vi "Example - Download with Progress and Abort.vi"() -> ()   [LabVIEW 2019]
uses:
  <vilib>/httpClient/LabVIEWHTTPClient.lvlib
  Get Async.lvlib
  <vilib>/Utility/sysdir.llb/System Directory Type.ctl
  HTTP Client Extensions.lvlib
panel:
  out "Rediect URLs":string[](array[string])
  in  "timeout (10000)":i32=10000
  out "complete":bool[](array[boolean])
  in  "Exit":bool
  in  "Start":bool
  in  "Files to Download":string[](array[string])=["http://download.ni.com/evaluation/labview/lvtn/vipm/packages/NI_GDS_2016/NI_GDS_2016-1.1.83.83.vip", "http://download.ni.com/evaluation/labview/lvtn/vipm/packages/ni_gds/ni_gds-1.1.87.94.vip", "http://download.ni.com/evaluation/labview/lvtn/vipm/packages/s5s_aloha/s5s_aloha-2.0.0.22.vip", "http://download.ni.com/evaluation/labview/lvtn/vipm/packages/s5s_aloha_system/s5s_aloha_system-2.0.0.22.vip"]
  out "Progress":dbl[](array[slide]) scale=0.0..100.0
  out "bytes downloaded":i64[](array[numeric])
  out "file size (bytes)":i64[](array[numeric])
  in  "Abort":bool
  in  "Folder to save file(s)":path
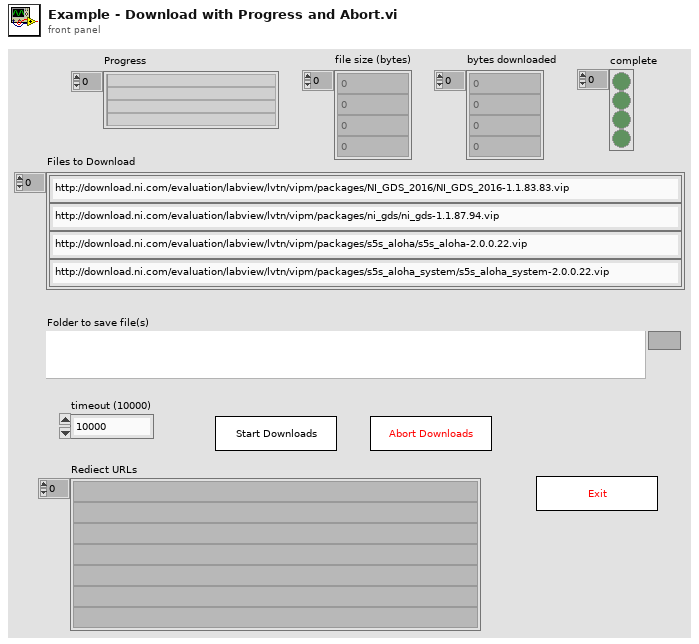
[diagram p1: front panel]
types:
  T1 = typedef "System Directory Type.ctl" = i32
  T2 = typedef "LabVIEWHTTPClient.lvlib/ClientHandle.ctl" = refnum<k1>
  T3 = typedef "HTTP Client Extensions.lvlib/Get Async.lvlib/Refnum Type.ctl" = refnum<k1>
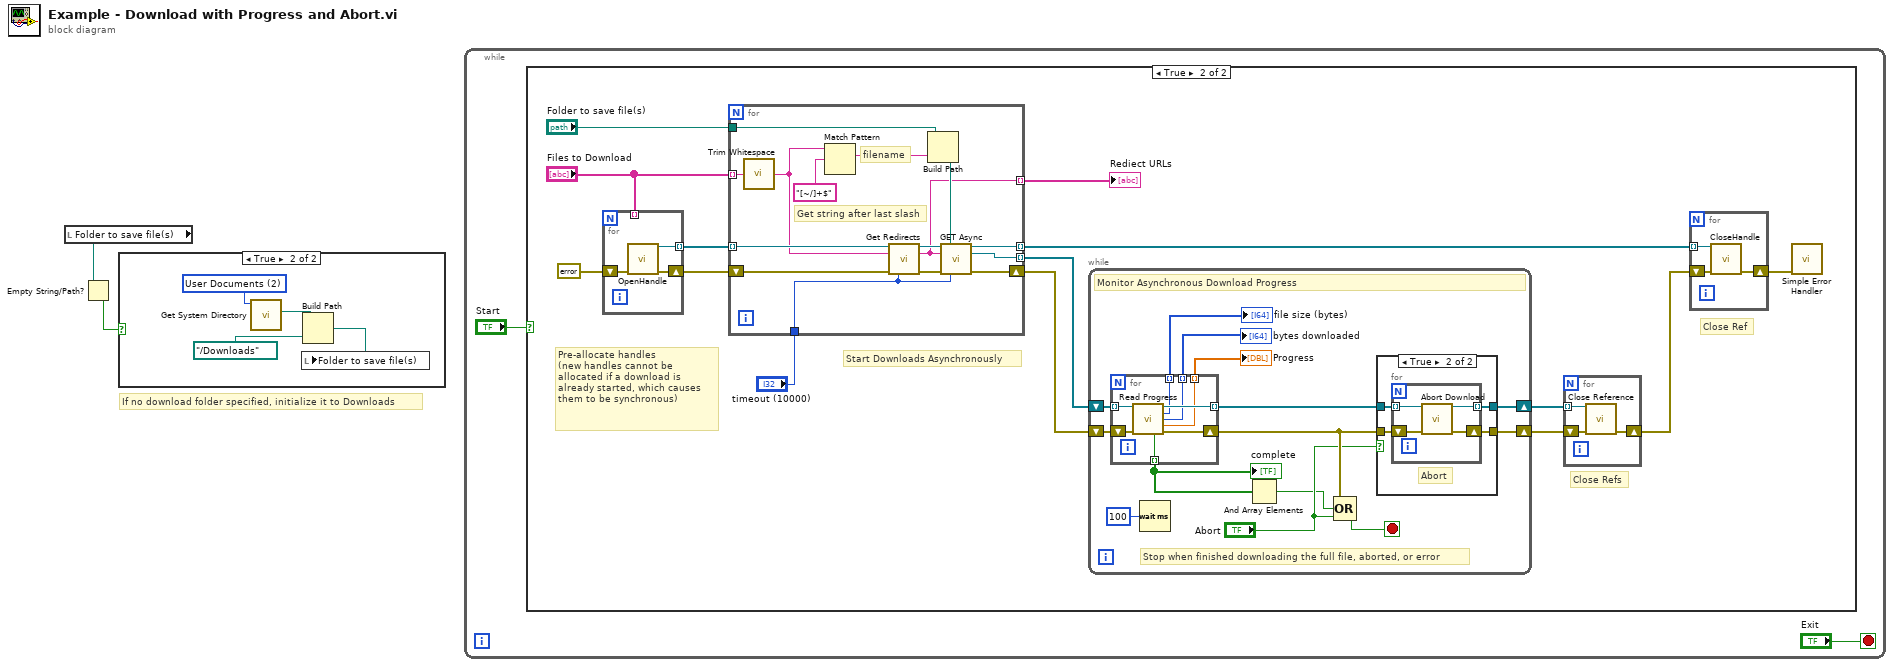
[diagram p0: block diagram]
diagram:
  # "If no download folder specified, initialize it to Downloads"
  n1 = local read "Folder to save file(s)"() -> (w2:path)
  n2 = Empty String/Path?(string/path=w2) -> (empty?=w1:bool)
  n3 = case shown="True" w1 {
    frame False {
    }
    frame True {
      w6 = T1 2 items=["User Home"=0, "User Desktop"=1, "User Documents"=2, "User Application Data"=3, "User Preferences"=4, "User Temporary"=5, "Public Documents"=6, "Public Application Data"=7, "Public Preferences"=8, "Public Cache"=13, "System Core Libraries"=9, "System Installed Libraries"=10, "Application Files"=11, "Boot Volume Root"=12] ("system directory type")
      n4 = call <vilib>:"Get System Directory.vi"("system directory type"=w6) -> ("system directory"=w5:path)  [unwired: 10 in]
      n5 = Build Path(base path=w5, name or relative path=path "../Downloads" ("base path")) -> (appended path=w3:path)
      n6 = local write "Folder to save file(s)"(w3) -> ()
    }
  }
  n7 = while {
    stop <- "Exit" stop-if-true
    n8 = case shown="True" "Start" {
      frame False {
      }
      frame True {
        # "Start Downloads Asynchronously"
        # "Close Ref"
        # "Close Refs"
        # "Pre-allocate handles\n(new handles cannot be allocated if a download is already started, which causes them to be synchronous)"
        n9 = for {
          shift-right: [w24] -> w14
          shift-left: errorcluster {"status"=FALSE, "code"=0, "source"=""} ("error out") -> [w25]
          tunnel: [w23] -> w13 mode=indexing
          tunnel: "Files to Download" -> [_] mode=indexing
          n10 = call <vilib>:"OpenHandle.vi"("error in (no error)"=w25) -> ("client handle out"=w23:T2, "error out"=w24:errorcluster)  [unwired: 13 in]
        }
        n11 = for {
          tunnel: "Folder to save file(s)" -> [w44]
          tunnel: [w41] -> w16 mode=indexing
          tunnel: "Files to Download" -> [w39] mode=indexing
          shift-right: [w42] -> w21
          shift-left: w14 -> [w34]
          tunnel: [w40] -> w20 mode=indexing
          tunnel: w13 -> [w37] mode=indexing
          tunnel: "timeout (10000)" -> [w33]
          tunnel: [w32] -> w9 mode=indexing
          # "Get string after last slash"
          # "filename"
          n12 = call <vilib>:"Trim Whitespace.vi"("string"=w39) -> ("trimmed string"=w36:string)  [unwired: 1 in]
          n13 = Match Pattern(string=w36, regular expression="[~/]+$") -> (match substring=w45:string)  [unwired: 1 in, 3 out]
          n14 = call "Get Redirects.vi"("client handle"=w37, "url"=w36, "error in (no error)"=w34, "timeout (10000)"=w33) -> ("client handle out"=w38:T2, "url out"=w32:string, "error out"=w35:errorcluster)  [unwired: 5 in, 4 out]
          n15 = Build Path(base path=w44, name or relative path=w45) -> (appended path=w43:path)
          n16 = call "GET Async.vi"("client handle"=w38, "output file"=w43, "url"=w32, "error in (no error)"=w35, "timeout (10000)"=w33) -> ("client handle out"=w40:T2, "get async handle"=w41:T3, "error out"=w42:errorcluster)  [unwired: 7 in, 1 out]
        }
        "Rediect URLs" <- w9
        n17 = while {
          shift-right: [w57] -> w18
          shift-left: w21 -> [w58]
          shift-right: [w53] -> w19
          shift-left: w16 -> [w59]
          stop <- w60 stop-if-true
          # "Stop when finished downloading the full file, aborted, or error"
          # "Monitor Asynchronous Download Progress"
          n18 = for {
            tunnel: w59 -> [w68] mode=indexing
            tunnel: [w61] -> w52 mode=indexing
            tunnel: [w62] -> w51 mode=indexing
            tunnel: [w65] -> w54 mode=indexing
            tunnel: [w64] -> w48 mode=indexing
            tunnel: [w63] -> w50 mode=indexing
            shift-right: [w66] -> w56
            shift-left: w58 -> [w67]
            n19 = call "Read Progress.vi"("HTTP GET Async handle"=w68, "error in (no error)"=w67) -> ("HTTP GET Async handle out"=w65:T3, "file size"=w62:i64, "bytes downloaded"=w61:i64, "percent complete"=w64:dbl, "download complete"=w63:bool, "error out"=w66:errorcluster)  [unwired: 8 in]
          }
          "bytes downloaded" <- w52
          "file size (bytes)" <- w51
          "Progress" <- w48
          "complete" <- w50
          n20 = Wait (ms)(milliseconds to wait=u32 100) -> ()  [unwired: 1 out]
          n21 = And Array Elements(Boolean array=w50) -> (logical AND=w49:bool)
          n22 = Compound Arithmetic op=OR(w56, w49, "Abort") -> (w60:bool)
          n23 = case shown="True" "Abort" {
            tunnel: [w70 w74] -> w57
            tunnel: w56 -> [w70 w73]
            tunnel: w54 -> [w69 w72]
            tunnel: [w69 w71] -> w53
            frame False {
            }
            frame True {
              # "Abort"
              n24 = for {
                shift-right: [w78] -> w74
                shift-left: w73 -> [w77]
                tunnel: w72 -> [w76] mode=indexing
                tunnel: [w75] -> w71 mode=indexing
                n25 = call "Abort Download.vi"("HTTP GET Async handle"=w76, "error in (no error)"=w77) -> ("HTTP GET Async handle out"=w75:T3, "error out"=w78:errorcluster)  [unwired: 12 in]
              }
            }
          }
        }
        n26 = for {
          tunnel: w19 -> [w31] mode=indexing
          shift-right: [w29] -> w17
          shift-left: w18 -> [w30]
          n27 = call "Close Reference.vi"("HTTP GET Async handle"=w31, "error in (no error)"=w30) -> ("error out"=w29:errorcluster)  [unwired: 13 in]
        }
        n28 = for {
          tunnel: w20 -> [w27] mode=indexing
          shift-right: [w28] -> w11
          shift-left: w17 -> [w26]
          n29 = call <vilib>:"CloseHandle.vi"("client handle"=w27, "error in (no error)"=w26) -> ("error out"=w28:errorcluster)  [unwired: 13 in]
        }
        n30 = call <vilib>:"Simple Error Handler.vi"("error in (no error)"=w11) -> ()  [unwired: 4 in, 5 out]
      }
    }
  }
